vi "Wheel of Doom Simulation.vi"() -> ()   [LabVIEW 2019]
uses:
  <extravilib>/ChannelInstances/Tag-dbl/Write With Abort.vi
  <extravilib>/ChannelInstances/Tag-dbl/Read With Abort.vi
  <extravilib>/ChannelInstances/Tag-dbl/Instantiate.vi
  <extravilib>/ChannelInstances/Tag-dbl/EndpointRead.vi
  <extravilib>/ChannelInstances/Tag-dbl/Endpoint.vi
  <vilib>/ptbypt/NI_PtbyPt.lvlib
  <extravilib>/ChannelInstances/Tag-dbl.lvlib
panel:
  in  "Mag Sensor Hysteresis":dbl
  in  "Mag Sensor Location [0 60]":dbl
  out "Sensor Data":i16(graph)
  in  "Control":bool[](array[boolean])
  out "Array":bool[](array[boolean])
  out "Wheel of Doom":T1(knob)={"Numeric"=0.0, "Numeric"=52.26969305988342, "Numeric"=96.7671113931624, "Numeric"=132.3047891851368, "Numeric"=227.24522261170432, "Numeric"=300.09363485419897, "Numeric"=28.56852087951421, "Numeric"=88.15896511134666, "Numeric"=149.36175476175384, "Numeric"=211.20095574850066, "Numeric"=272.8635678940626, "Numeric"=330.74842972211724} scale=0.0..360.0
  in  "RPM":dbl=1.0 format="%0.2f"
  # "Controls"
  # "Settings"
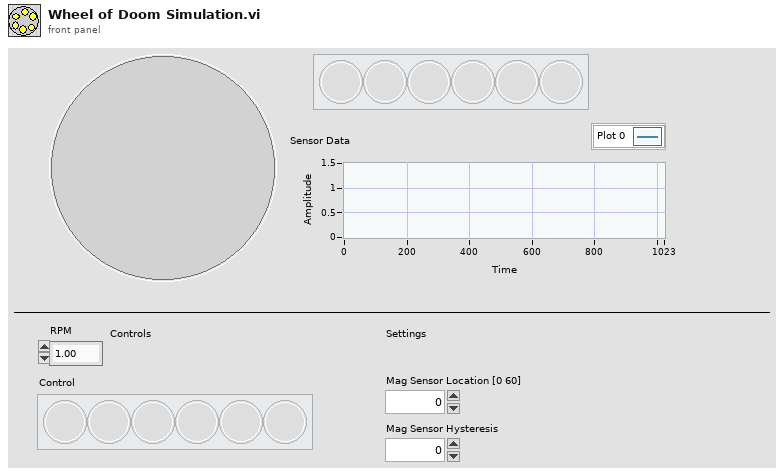
[diagram p1: front panel]
types:
  T1 = cluster{"Numeric":dbl, "Numeric":dbl, "Numeric":dbl, "Numeric":dbl, "Numeric":dbl, "Numeric":dbl, "Numeric":dbl, "Numeric":dbl, "Numeric":dbl, "Numeric":dbl, "Numeric":dbl, "Numeric":dbl}
  T2 = typedef "Tag-dbl.lvlib/))Channel.ctl" = refnum<queue>
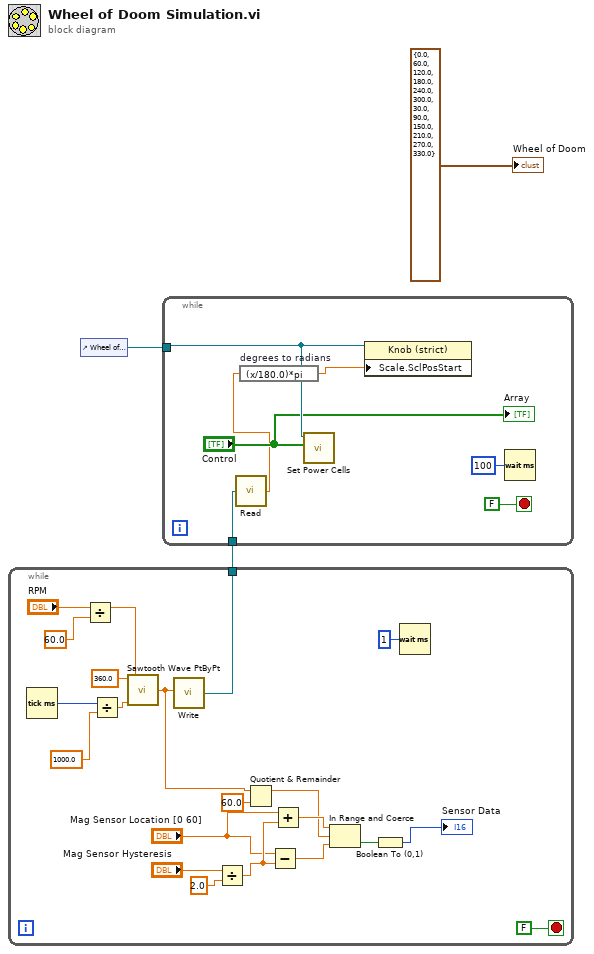
[diagram p0: block diagram]
diagram:
  n1 = while {
    tunnel: [w5] -> w2
    stop <- FALSE stop-if-true
    n2 = Tick Count (ms)() -> (millisecond timer value=w12:u32)
    n3 = Divide(x="RPM", y=60.0 ("x")) -> (x/y=w14:dbl)
    n4 = Divide(x=w12, y=1000.0) -> (x/y=w11:dbl)
    n5 = call <vilib>:"Sawtooth Wave PtByPt.vi"("time"=w11, "frequency"=w14, "amplitude"=360.0) -> ("sawtooth wave"=w8:dbl)  [unwired: 1 in]
    n6 = call <extravilib>:"Write.vi"("element"=w8) -> ("channel"=w5:T2)  [unwired: 1 out]
    n7 = Divide(x="Mag Sensor Hysteresis", y=2.0) -> (x/y=w21:dbl)
    n8 = Quotient & Remainder(x=w8, y=60.0) -> (x-y*floor(x/y)=w4:dbl)  [unwired: 1 out]
    n9 = Subtract(x="Mag Sensor Location [0 60]", y=w21) -> (x-y=w23:dbl)
    n10 = Add(x="Mag Sensor Location [0 60]", y=w21) -> (x+y=w22:dbl)
    n11 = In Range and Coerce(upper limit=w22, x=w4, lower limit=w23) -> (In Range?=w16:bool)  [unwired: 1 out]
    n12 = Boolean To (0,1)(Boolean=w16) -> (0, 1=→"Sensor Data":i16)
    n13 = Wait (ms)(milliseconds to wait=u32 1) -> ()  [unwired: 1 out]
  }
  n14 = control-ref of="Wheel of Doom"() -> (w3:refnum<vi>)
  n15 = while {
    tunnel: w3 -> [w29]
    tunnel: w2 -> [w26]
    stop <- FALSE stop-if-true
    n16 = call <extravilib>:"Read.vi"("channel"=w26) -> ("element"=w25:dbl)  [unwired: 1 in, 1 out]
    n17 = expression code="(x/180.0)*pi" "degrees to radians"(w25) -> (w27:dbl)
    n18 = call "Set Power Cells.vi"("Array"="Control", "Knob in"=w29) -> ()  [unwired: 9 in, 1 out]
    n19 = property on="Property Node" class="Knob (strict)"(reference=w29, "Scale.SclPosStart"=w27) -> ()  [unwired: 1 in, 2 out]
    n20 = Wait (ms)(milliseconds to wait=u32 100) -> ()  [unwired: 1 out]
    "Array" <- "Control"
  }
  "Wheel of Doom" <- T1 {"Numeric"=0.0, "Numeric"=60.0, "Numeric"=120.0, "Numeric"=180.0, "Numeric"=240.0, "Numeric"=300.0, "Numeric"=30.0, "Numeric"=90.0, "Numeric"=150.0, "Numeric"=210.0, "Numeric"=270.0, "Numeric"=330.0} ("Wheel of Doom")
